vi "CreateModuleFile.vi"(8 "error in (no error)":errorcluster, 11 "PythonWrapper in":refnum<class "PythonWrapper.lvclass">) -> (0 "error out":errorcluster, 3 "PythonWrapper out":refnum<class "PythonWrapper.lvclass">)   [LabVIEW 2022 SP3, in "PythonWrapper.lvlib" / "PythonWrapper.lvclass"]
uses:
  PythonWrapper.lvclass
  PythonWrapper.lvclass/PythonWrapper.ctl
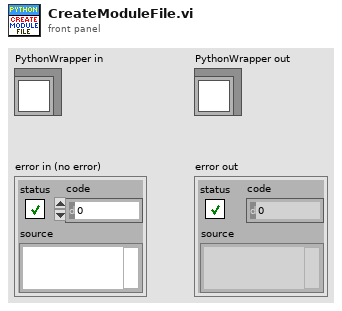
[diagram p1: front panel]
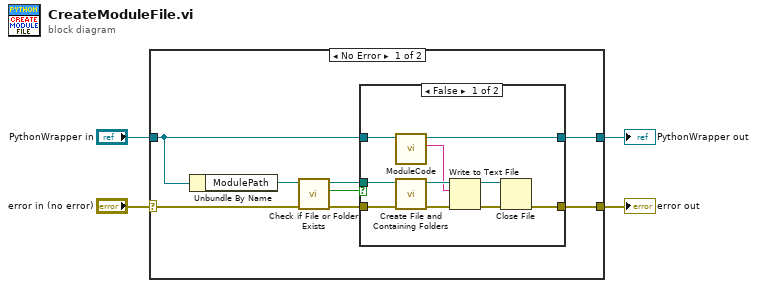
[diagram p0: block diagram]
diagram:
  n1 = case shown="No Error" "error in (no error)" {
    selector: "error in (no error)" -> [w11 w26]
    tunnel: [w10 w26] -> w3
    tunnel: "PythonWrapper in" -> [w5 w25]
    tunnel: [w6 w25] -> w1
    frame No Error {
      n2 = Unbundle By Name(w5) -> ("ModulePath"=w12:path)
      n3 = call <vilib>:"Check if File or Folder Exists.vi"("error in (no error)"=w11, "path"=w12) -> ("error out"=w9:errorcluster, "file or folder exists?"=w8:bool, "dup path"=w7:path)  [unwired: 7 in]
      n4 = case shown="False" w8 {
        tunnel: [w14 w24] -> w10
        tunnel: w9 -> [w21 w24]
        tunnel: w7 -> [w20 _]
        tunnel: [w16 w23] -> w6
        tunnel: w5 -> [w22 w23]
        frame False {
          n5 = call-dynamic "ModuleCode.vi"("PythonWrapper in"=w22) -> ("PythonCode"=w15:string, "PythonWrapper out"=w16:refnum<class "PythonWrapper.lvclass">)  [unwired: 9 in]
          n6 = call <vilib>:"Create File and Containing Folders.vi"("error in (no error)"=w21, "file path"=w20) -> ("error out"=w19:errorcluster, "refnum out"=w17:refnum<file>)  [unwired: 8 in]
          n7 = Write to Text File(file (use dialog)=w17, text=w15, error in=w19) -> (refnum out=w13:refnum<file>, error out=w18:errorcluster)  [unwired: 1 in, 1 out]
          n8 = Close File(refnum=w13, error in=w18) -> (error out=w14:errorcluster)  [unwired: 1 out]
        }
        frame True {
        }
      }
    }
    frame Error {
    }
  }
  "error out" <- w3
  "PythonWrapper out" <- w1
